vi "Test Expt Variables Fast Query.vi"() -> ()   [LabVIEW 2013]
panel:
  out "error out":errorcluster
  out "data":string[][](array[string])
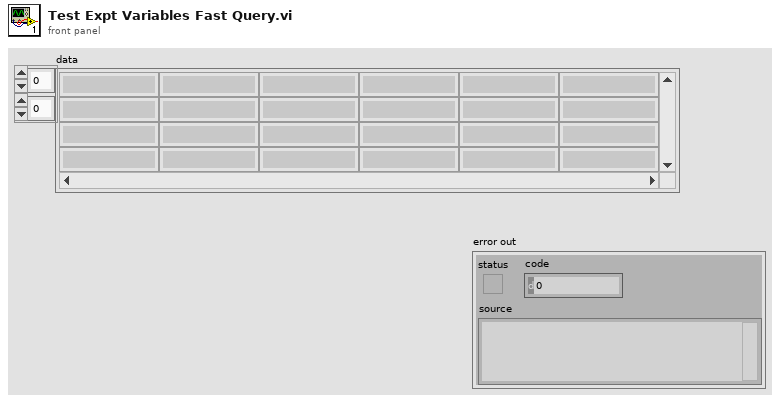
[diagram p1: front panel]
types:
  T1 = typedef "mysql_authentication.ctl" = cluster{"User":string, "Password":string, "Database":string}
  T2 = cluster{"Port":u16, "IP Address":string, "Authentication":T1}
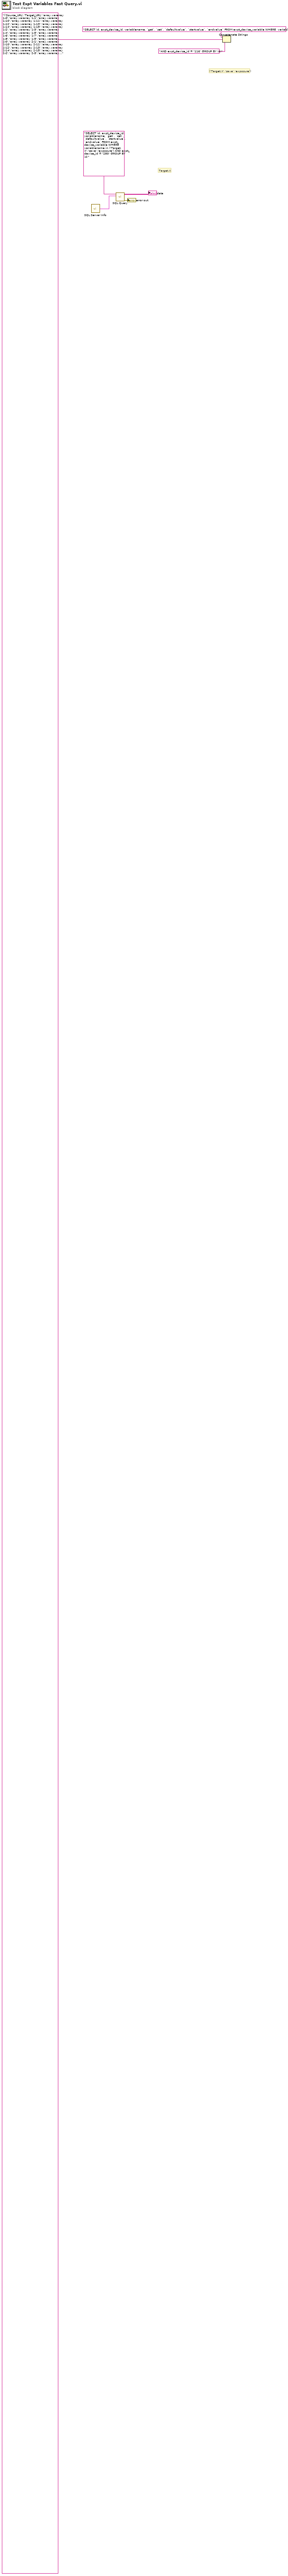
[diagram p0: block diagram]
diagram:
  # "('Target.X','save','exposure')"
  # "Target.X"
  n1 = call "SQL Server Info.vi"() -> ("SQL Server Info"=w7:T2)
  n2 = call "SQL Query.vi"("SQL Server Info"=w7, "Query"="SELECT id, expt_device_id, variablename, `get`, `set`, `defaultvalue`, `startvalue`, `endvalue` FROM expt_device_variable WHERE  variablename in ('Target.X','save','exposure') AND expt_device_id = '280' GROUP BY id;") -> ("error out"=→"error out":errorcluster, "data"=→"data":string[][])  [unwired: 8 in]
  n3 = Concatenate Strings("SELECT id, expt_device_id, variablename, `get`, `set`, `defaultvalue`, `startvalue`, `endvalue` FROM expt_device_variable WHERE  variablename in ", "('Source_URL','Target_URL','array.vararray 1-0','array.vararray 1-1','array.vararray 1-10','array.vararray 1-11','array.vararray 1-12','array.vararray 1-13','array.vararray 1-14','array.vararray 1-15','array.vararray 1-2','array.vararray 1-3','array.vararray 1-4','array.vararray 1-5','array.vararray 1-6','array.vararray 1-7','array.vararray 1-8','array.vararray 1-9','array.vararray 2-0','array.vararray 2-1','array.vararray 2-10','array.vararray 2-11','array.vararray 2-12','array.vararray 2-13','array.vararray 2-14','array.vararray 2-15','array.vararray 2-2','array.vararray 2-3','array.vararray 2-5','array.vararray 2-7','array.vararray 2-8','array.vararray 2-9','array.vararray 3-0','array.vararray 3-1','array.vararray 3-10','array.vararray 3-11','array.vararray 3-12','array.vararray 3-13','array.vararray 3-14','array.vararray 3-15','array.vararray 3-2','array.vararray 3-3','array.vararray 3-4','array.vararray 3-5','array.vararray 3-6','array.vararray 3-7','array.vararray 3-8','array.vararray 3-9','array.vararray 4-0','array.vararray 4-1','array.vararray 4-10','array.vararray 4-11','array.vararray 4-12','array.vararray 4-13','array.vararray 4-14','array.vararray 4-15','array.vararray 4-2','array.vararray 4-3','array.vararray 4-4','array.vararray 4-5','array.vararray 4-6','array.vararray 4-7','array.vararray 4-8','array.vararray 4-9','array.vararray 2-4','array.vararray 2-6','index.varindex 1-0','index.varindex 1-1','index.varindex 1-10','index.varindex 1-11','index.varindex 1-12','index.varindex 1-13','index.varindex 1-14','index.varindex 1-15','index.varindex 1-2','index.varindex 1-3','index.varindex 1-4','index.varindex 1-5','index.varindex 1-6','index.varindex 1-7','index.varindex 1-8','index.varindex 1-9','index.varindex 2-0','index.varindex 2-1','index.varindex 2-10','index.varindex 2-11','index.varindex 2-12','index.varindex 2-13','index.varindex 2-14','index.varindex 2-15','index.varindex 2-2','index.varindex 2-3','index.varindex 2-4','index.varindex 2-5','index.varindex 2-6','index.varindex 2-7','index.varindex 2-8','index.varindex 2-9','index.varindex 3-0','index.varindex 3-1','index.varindex 3-10','index.varindex 3-11','index.varindex 3-12','index.varindex 3-13','index.varindex 3-14','index.varindex 3-15','index.varindex 3-2','index.varindex 3-3','index.varindex 3-4','index.varindex 3-5','index.varindex 3-6','index.varindex 3-7','index.varindex 3-8','index.varindex 3-9','index.varindex 4-0','index.varindex 4-1','index.varindex 4-10','index.varindex 4-11','index.varindex 4-12','index.varindex 4-13','index.varindex 4-14','index.varindex 4-15','index.varindex 4-2','index.varindex 4-3','index.varindex 4-4','index.varindex 4-5','index.varindex 4-6','index.varindex 4-7','index.varindex 4-8','index.varindex 4-9','name.var 1-0','name.var 1-1','name.var 1-10','name.var 1-11','name.var 1-12','name.var 1-13','name.var 1-14','name.var 1-15','name.var 1-3','name.var 1-4','name.var 1-5','name.var 1-6','name.var 1-7','name.var 1-8','name.var 1-9','name.var 2-0','name.var 2-1','name.var 2-10','name.var 2-11','name.var 2-12','name.var 2-13','name.var 2-14','name.var 2-15','name.var 2-3','name.var 2-4','name.var 2-5','name.var 2-6','name.var 2-7','name.var 2-8','name.var 2-9','name.var 3-0','name.var 3-1','name.var 3-10','name.var 3-11','name.var 3-12','name.var 3-13','name.var 3-14','name.var 3-15','name.var 3-3','name.var 3-4','name.var 3-5','name.var 3-6','name.var 3-7','name.var 3-8','name.var 3-9','name.var 4-0','name.var 4-1','name.var 4-10','name.var 4-11','name.var 4-12','name.var 4-13','name.var 4-14','name.var 4-15','name.var 4-3','name.var 4-4','name.var 4-5','name.var 4-6','name.var 4-7','name.var 4-8','name.var 4-9','statusboolarray1.var 1-0','statusboolarray1.var 1-1','statusboolarray1.var 1-10','statusboolarray1.var 1-11','statusboolarray1.var 1-12','statusboolarray1.var 1-13','statusboolarray1.var 1-14','statusboolarray1.var 1-15','statusboolarray1.var 1-2','statusboolarray1.var 1-3','statusboolarray1.var 1-4','statusboolarray1.var 1-5','statusboolarray1.var 1-6','statusboolarray1.var 1-7','statusboolarray1.var 1-8','statusboolarray1.var 1-9','statusboolarray1.var 2-0','statusboolarray1.var 2-1','statusboolarray1.var 2-10','statusboolarray1.var 2-11','statusboolarray1.var 2-12','statusboolarray1.var 2-13','statusboolarray1.var 2-14','statusboolarray1.var 2-15','statusboolarray1.var 2-2','statusboolarray1.var 2-3','statusboolarray1.var 2-4','statusboolarray1.var 2-5','statusboolarray1.var 2-6','statusboolarray1.var 2-7','statusboolarray1.var 2-8','statusboolarray1.var 2-9','statusboolarray1.var 3-0','statusboolarray1.var 3-1','statusboolarray1.var 3-10','statusboolarray1.var 3-11','statusboolarray1.var 3-12','statusboolarray1.var 3-13','statusboolarray1.var 3-14','statusboolarray1.var 3-15','statusboolarray1.var 3-2','statusboolarray1.var 3-3','statusboolarray1.var 3-4','statusboolarray1.var 3-5','statusboolarray1.var 3-6','statusboolarray1.var 3-7','statusboolarray1.var 3-8','statusboolarray1.var 3-9','statusboolarray1.var 4-0','statusboolarray1.var 4-1','statusboolarray1.var 4-10','statusboolarray1.var 4-11','statusboolarray1.var 4-12','statusboolarray1.var 4-13','statusboolarray1.var 4-14','statusboolarray1.var 4-15','statusboolarray1.var 4-2','statusboolarray1.var 4-3','statusboolarray1.var 4-4','statusboolarray1.var 4-5','statusboolarray1.var 4-6','statusboolarray1.var 4-7','statusboolarray1.var 4-8','statusboolarray1.var 4-9','statusboolarray2.var 1-0','statusboolarray2.var 1-1','statusboolarray2.var 1-10','statusboolarray2.var 1-11','statusboolarray2.var 1-12','statusboolarray2.var 1-13','statusboolarray2.var 1-14','statusboolarray2.var 1-15','statusboolarray2.var 1-2','statusboolarray2.var 1-3','statusboolarray2.var 1-4','statusboolarray2.var 1-5','statusboolarray2.var 1-6','statusboolarray2.var 1-7','statusboolarray2.var 1-8','statusboolarray2.var 1-9','statusboolarray2.var 2-0','statusboolarray2.var 2-1','statusboolarray2.var 2-10','statusboolarray2.var 2-11','statusboolarray2.var 2-12','statusboolarray2.var 2-13','statusboolarray2.var 2-14','statusboolarray2.var 2-15','statusboolarray2.var 2-2','statusboolarray2.var 2-3','statusboolarray2.var 2-4','statusboolarray2.var 2-5','statusboolarray2.var 2-6','statusboolarray2.var 2-7','statusboolarray2.var 2-8','statusboolarray2.var 2-9','statusboolarray2.var 3-0','statusboolarray2.var 3-1','statusboolarray2.var 3-10','statusboolarray2.var 3-11','statusboolarray2.var 3-12','statusboolarray2.var 3-13','statusboolarray2.var 3-14','statusboolarray2.var 3-15','statusboolarray2.var 3-2','statusboolarray2.var 3-3','statusboolarray2.var 3-4','statusboolarray2.var 3-5','statusboolarray2.var 3-6','statusboolarray2.var 3-7','statusboolarray2.var 3-8','statusboolarray2.var 3-9','statusboolarray2.var 4-0','statusboolarray2.var 4-1','statusboolarray2.var 4-10','statusboolarray2.var 4-11','statusboolarray2.var 4-12','statusboolarray2.var 4-13','statusboolarray2.var 4-14','statusboolarray2.var 4-15','statusboolarray2.var 4-2','statusboolarray2.var 4-3','statusboolarray2.var 4-4','statusboolarray2.var 4-5','statusboolarray2.var 4-6','statusboolarray2.var 4-7','statusboolarray2.var 4-8','statusboolarray2.var 4-9','statusboolarray3.var 1-0','statusboolarray3.var 1-1','statusboolarray3.var 1-10','statusboolarray3.var 1-11','statusboolarray3.var 1-12','statusboolarray3.var 1-13','statusboolarray3.var 1-14','statusboolarray3.var 1-15','statusboolarray3.var 1-2','statusboolarray3.var 1-3','statusboolarray3.var 1-4','statusboolarray3.var 1-5','statusboolarray3.var 1-6','statusboolarray3.var 1-7','statusboolarray3.var 1-8','statusboolarray3.var 1-9','statusboolarray3.var 2-0','statusboolarray3.var 2-1','statusboolarray3.var 2-10','statusboolarray3.var 2-11','statusboolarray3.var 2-12','statusboolarray3.var 2-13','statusboolarray3.var 2-14','statusboolarray3.var 2-15','statusboolarray3.var 2-2','statusboolarray3.var 2-3','statusboolarray3.var 2-4','statusboolarray3.var 2-5','statusboolarray3.var 2-6','statusboolarray3.var 2-7','statusboolarray3.var 2-8','statusboolarray3.var 2-9','statusboolarray3.var 3-0','statusboolarray3.var 3-1','statusboolarray3.var 3-10','statusboolarray3.var 3-11','statusboolarray3.var 3-12','statusboolarray3.var 3-13','statusboolarray3.var 3-14','statusboolarray3.var 3-15','statusboolarray3.var 3-2','statusboolarray3.var 3-3','statusboolarray3.var 3-4','statusboolarray3.var 3-5','statusboolarray3.var 3-6','statusboolarray3.var 3-7','statusboolarray3.var 3-8','statusboolarray3.var 3-9','statusboolarrayname1.var 1-0','statusboolarrayname1.var 1-1','statusboolarrayname1.var 1-10','statusboolarrayname1.var 1-11','statusboolarrayname1.var 1-12','statusboolarrayname1.var 1-13','statusboolarrayname1.var 1-14','statusboolarrayname1.var 1-15','statusboolarrayname1.var 1-3','statusboolarrayname1.var 1-4','statusboolarrayname1.var 1-5','statusboolarrayname1.var 1-6','statusboolarrayname1.var 1-7','statusboolarrayname1.var 1-8','statusboolarrayname1.var 1-9','statusboolarrayname1.var 2-0','statusboolarrayname1.var 2-1','statusboolarrayname1.var 2-10','statusboolarrayname1.var 2-11','statusboolarrayname1.var 2-12','statusboolarrayname1.var 2-13','statusboolarrayname1.var 2-14','statusboolarrayname1.var 2-15','statusboolarrayname1.var 2-3','statusboolarrayname1.var 2-4','statusboolarrayname1.var 2-5','statusboolarrayname1.var 2-6','statusboolarrayname1.var 2-7','statusboolarrayname1.var 2-8','statusboolarrayname1.var 2-9','statusboolarrayname1.var 3-0','statusboolarrayname1.var 3-1','statusboolarrayname1.var 3-10','statusboolarrayname1.var 3-11','statusboolarrayname1.var 3-12','statusboolarrayname1.var 3-13','statusboolarrayname1.var 3-14','statusboolarrayname1.var 3-15','statusboolarrayname1.var 3-3','statusboolarrayname1.var 3-4','statusboolarrayname1.var 3-5','statusboolarrayname1.var 3-6','statusboolarrayname1.var 3-7','statusboolarrayname1.var 3-8','statusboolarrayname1.var 3-9','statusboolarrayname1.var 4-0','statusboolarrayname1.var 4-1','statusboolarrayname1.var 4-10','statusboolarrayname1.var 4-11','statusboolarrayname1.var 4-12','statusboolarrayname1.var 4-13','statusboolarrayname1.var 4-14','statusboolarrayname1.var 4-15','statusboolarrayname1.var 4-3','statusboolarrayname1.var 4-4','statusboolarrayname1.var 4-5','statusboolarrayname1.var 4-6','statusboolarrayname1.var 4-7','statusboolarrayname1.var 4-8','statusboolarrayname1.var 4-9','statusboolarrayname2.var 1-0','statusboolarrayname2.var 1-1','statusboolarrayname2.var 1-10','statusboolarrayname2.var 1-11','statusboolarrayname2.var 1-12','statusboolarrayname2.var 1-13','statusboolarrayname2.var 1-14','statusboolarrayname2.var 1-15','statusboolarrayname2.var 1-3','statusboolarrayname2.var 1-4','statusboolarrayname2.var 1-5','statusboolarrayname2.var 1-6','statusboolarrayname2.var 1-7','statusboolarrayname2.var 1-8','statusboolarrayname2.var 1-9','statusboolarrayname2.var 2-0','statusboolarrayname2.var 2-1','statusboolarrayname2.var 2-10','statusboolarrayname2.var 2-11','statusboolarrayname2.var 2-12','statusboolarrayname2.var 2-13','statusboolarrayname2.var 2-14','statusboolarrayname2.var 2-15','statusboolarrayname2.var 2-3','statusboolarrayname2.var 2-4','statusboolarrayname2.var 2-5','statusboolarrayname2.var 2-6','statusboolarrayname2.var 2-7','statusboolarrayname2.var 2-8','statusboolarrayname2.var 2-9','statusboolarrayname2.var 3-0','statusboolarrayname2.var 3-1','statusboolarrayname2.var 3-10','statusboolarrayname2.var 3-11','statusboolarrayname2.var 3-12','statusboolarrayname2.var 3-13','statusboolarrayname2.var 3-14','statusboolarrayname2.var 3-15','statusboolarrayname2.var 3-3','statusboolarrayname2.var 3-4','statusboolarrayname2.var 3-5','statusboolarrayname2.var 3-6','statusboolarrayname2.var 3-7','statusboolarrayname2.var 3-8','statusboolarrayname2.var 3-9','statusboolarrayname2.var 4-0','statusboolarrayname2.var 4-1','statusboolarrayname2.var 4-10','statusboolarrayname2.var 4-11','statusboolarrayname2.var 4-12','statusboolarrayname2.var 4-13','statusboolarrayname2.var 4-14','statusboolarrayname2.var 4-15','statusboolarrayname2.var 4-3','statusboolarrayname2.var 4-4','statusboolarrayname2.var 4-5','statusboolarrayname2.var 4-6','statusboolarrayname2.var 4-7','statusboolarrayname2.var 4-8','statusboolarrayname2.var 4-9','statusboolarrayname3.var 1-0','statusboolarrayname3.var 1-1','statusboolarrayname3.var 1-10','statusboolarrayname3.var 1-11','statusboolarrayname3.var 1-12','statusboolarrayname3.var 1-13','statusboolarrayname3.var 1-14','statusboolarrayname3.var 1-15','statusboolarrayname3.var 1-3','statusboolarrayname3.var 1-4','statusboolarrayname3.var 1-5','statusboolarrayname3.var 1-6','statusboolarrayname3.var 1-7','statusboolarrayname3.var 1-8','statusboolarrayname3.var 1-9','statusboolarrayname3.var 2-0','statusboolarrayname3.var 2-1','statusboolarrayname3.var 2-10','statusboolarrayname3.var 2-11','statusboolarrayname3.var 2-12','statusboolarrayname3.var 2-13','statusboolarrayname3.var 2-14','statusboolarrayname3.var 2-15','statusboolarrayname3.var 2-3','statusboolarrayname3.var 2-4','statusboolarrayname3.var 2-5','statusboolarrayname3.var 2-6','statusboolarrayname3.var 2-7','statusboolarrayname3.var 2-8','statusboolarrayname3.var 2-9','statusboolarrayname3.var 3-0','statusboolarrayname3.var 3-1','statusboolarrayname3.var 3-10','statusboolarrayname3.var 3-11','statusboolarrayname3.var 3-12','statusboolarrayname3.var 3-13','statusboolarrayname3.var 3-14','statusboolarrayname3.var 3-15','statusboolarrayname3.var 3-3','statusboolarrayname3.var 3-4','statusboolarrayname3.var 3-5','statusboolarrayname3.var 3-6','statusboolarrayname3.var 3-7','statusboolarrayname3.var 3-8','statusboolarrayname3.var 3-9','statusfloatarray.var 1-0','statusfloatarray.var 1-1','statusfloatarray.var 1-10','statusfloatarray.var 1-11','statusfloatarray.var 1-12','statusfloatarray.var 1-13','statusfloatarray.var 1-14','statusfloatarray.var 1-15','statusfloatarray.var 1-2','statusfloatarray.var 1-3','statusfloatarray.var 1-4','statusfloatarray.var 1-5','statusfloatarray.var 1-6','statusfloatarray.var 1-7','statusfloatarray.var 1-8','statusfloatarray.var 1-9','statusfloatarray.var 2-0','statusfloatarray.var 2-1','statusfloatarray.var 2-2','statusfloatarray.var 2-3','statusfloatarray.var 2-4','statusfloatarray.var 2-5','statusfloatarray.var 2-6','statusfloatarray.var 2-7','statusfloatarrayname.var 1-0','statusfloatarrayname.var 1-1','statusfloatarrayname.var 1-10','statusfloatarrayname.var 1-11','statusfloatarrayname.var 1-12','statusfloatarrayname.var 1-13','statusfloatarrayname.var 1-14','statusfloatarrayname.var 1-15','statusfloatarrayname.var 1-3','statusfloatarrayname.var 1-4','statusfloatarrayname.var 1-5','statusfloatarrayname.var 1-6','statusfloatarrayname.var 1-7','statusfloatarrayname.var 1-8','statusfloatarrayname.var 1-9','statusfloatarrayname.var 2-0','statusfloatarrayname.var 2-1','statusfloatarrayname.var 2-3','statusfloatarrayname.var 2-4','statusfloatarrayname.var 2-5','statusfloatarrayname.var 2-6','statusfloatarrayname.var 2-7','statusintegerarray.var 1-0','statusintegerarray.var 1-1','statusintegerarray.var 1-10','statusintegerarray.var 1-11','statusintegerarray.var 1-12','statusintegerarray.var 1-13','statusintegerarray.var 1-14','statusintegerarray.var 1-15','statusintegerarray.var 1-2','statusintegerarray.var 1-3','statusintegerarray.var 1-4','statusintegerarray.var 1-5','statusintegerarray.var 1-6','statusintegerarray.var 1-7','statusintegerarray.var 1-8','statusintegerarray.var 1-9','statusintegerarray.var 2-0','statusintegerarray.var 2-1','statusintegerarray.var 2-10','statusintegerarray.var 2-11','statusintegerarray.var 2-12','statusintegerarray.var 2-13','statusintegerarray.var 2-14','statusintegerarray.var 2-2','statusintegerarray.var 2-3','statusintegerarray.var 2-4','statusintegerarray.var 2-5','statusintegerarray.var 2-6','statusintegerarray.var 2-7','statusintegerarray.var 2-8','statusintegerarray.var 2-9','statusintegerarray.var 3-0','statusintegerarray.var 3-1','statusintegerarray.var 3-10','statusintegerarray.var 3-11','statusintegerarray.var 3-12','statusintegerarray.var 3-13','statusintegerarray.var 3-14','statusintegerarray.var 3-15','statusintegerarray.var 3-2','statusintegerarray.var 3-3','statusintegerarray.var 3-4','statusintegerarray.var 3-5','statusintegerarray.var 3-6','statusintegerarray.var 3-7','statusintegerarray.var 3-8','statusintegerarray.var 3-9','statusintegerarray.var 2-15','statusintegerarrayname.var 1-0','statusintegerarrayname.var 1-1','statusintegerarrayname.var 1-10','statusintegerarrayname.var 1-11','statusintegerarrayname.var 1-12','statusintegerarrayname.var 1-13','statusintegerarrayname.var 1-14','statusintegerarrayname.var 1-15','statusintegerarrayname.var 1-3','statusintegerarrayname.var 1-4','statusintegerarrayname.var 1-5','statusintegerarrayname.var 1-6','statusintegerarrayname.var 1-7','statusintegerarrayname.var 1-8','statusintegerarrayname.var 1-9','statusintegerarrayname.var 2-0','statusintegerarrayname.var 2-1','statusintegerarrayname.var 2-10','statusintegerarrayname.var 2-11','statusintegerarrayname.var 2-12','statusintegerarrayname.var 2-13','statusintegerarrayname.var 2-14','statusintegerarrayname.var 2-15','statusintegerarrayname.var 2-3','statusintegerarrayname.var 2-4','statusintegerarrayname.var 2-5','statusintegerarrayname.var 2-6','statusintegerarrayname.var 2-7','statusintegerarrayname.var 2-8','statusintegerarrayname.var 2-9','statusintegerarrayname.var 3-0','statusintegerarrayname.var 3-1','statusintegerarrayname.var 3-10','statusintegerarrayname.var 3-11','statusintegerarrayname.var 3-12','statusintegerarrayname.var 3-13','statusintegerarrayname.var 3-14','statusintegerarrayname.var 3-15','statusintegerarrayname.var 3-3','statusintegerarrayname.var 3-4','statusintegerarrayname.var 3-5','statusintegerarrayname.var 3-6','statusintegerarrayname.var 3-7','statusintegerarrayname.var 3-8','statusintegerarrayname.var 3-9','variable.var 1-0','variable.var 1-1','variable.var 1-10','variable.var 1-11','variable.var 1-12','variable.var 1-13','variable.var 1-14','variable.var 1-15','variable.var 1-2','variable.var 1-3','variable.var 1-4','variable.var 1-5','variable.var 1-6','variable.var 1-7','variable.var 1-8','variable.var 1-9','variable.var 2-0','variable.var 2-1','variable.var 2-10','variable.var 2-11','variable.var 2-12','variable.var 2-13','variable.var 2-14','variable.var 2-15','variable.var 2-2','variable.var 2-3','variable.var 2-4','variable.var 2-5','variable.var 2-6','variable.var 2-7','variable.var 2-8','variable.var 2-9','variable.var 3-0','variable.var 3-1','variable.var 3-10','variable.var 3-11','variable.var 3-12','variable.var 3-13','variable.var 3-14','variable.var 3-15','variable.var 3-2','variable.var 3-3','variable.var 3-4','variable.var 3-5','variable.var 3-6','variable.var 3-7','variable.var 3-8','variable.var 3-9','variable.var 4-0','variable.var 4-1','variable.var 4-10','variable.var 4-11','variable.var 4-12','variable.var 4-13','variable.var 4-14','variable.var 4-15','variable.var 4-2','variable.var 4-3','variable.var 4-4','variable.var 4-5','variable.var 4-6','variable.var 4-7','variable.var 4-8','variable.var 4-9','name.var 1-2','name.var 2-2','name.var 3-2','name.var 4-2','statusboolarrayname1.var 1-2','statusboolarrayname1.var 2-2','statusboolarrayname1.var 3-2','statusboolarrayname1.var 4-2','statusboolarrayname2.var 1-2','statusboolarrayname2.var 2-2','statusboolarrayname2.var 3-2','statusboolarrayname2.var 4-2','statusboolarrayname3.var 1-2','statusboolarrayname3.var 2-2','statusboolarrayname3.var 3-2','statusintegerarrayname.var 1-2','statusintegerarrayname.var 2-2','statusintegerarrayname.var 3-2','statusfloatarrayname.var 1-2','statusfloatarrayname.var 2-2') ", "AND expt_device_id = '116' GROUP BY id;" ("string")) -> ()  [unwired: 1 out]
